vi "saveBuildHeader_III.vi"(6 "No. Averages":i32, 7 "Filtering":bool, 9 "wl 3":string="445", 10 "wl in":string="377", 11 "wl1":string="320") -> (2 "wavelengths":string[](array[string]), 3 "header":string[](array[string]))   [LabVIEW 2011]
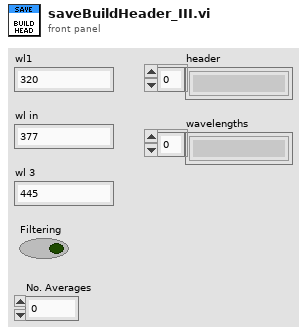
[diagram p1: front panel]
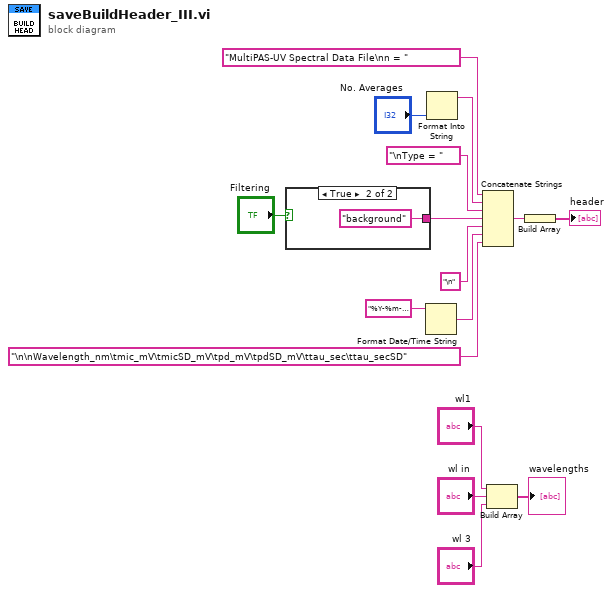
[diagram p0: block diagram]
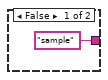
[diagram p2: hidden frame]
diagram:
  n1 = case shown="True" "Filtering" {
    tunnel: ["sample" "background"] -> w15
    frame False {
    }
    frame True {
    }
  }
  n2 = Format Date/Time String(time format string (%c)="%Y-%m-%d %H:%M:%S\t") -> (date/time string=w3:string)  [unwired: 2 in]
  n3 = Format Into String("No. Averages") -> (resulting string=w13:string)  [unwired: 3 in, 1 out]
  n4 = Concatenate Strings("MultiPAS-UV Spectral Data File\nn = ", w13, "\nType = " ("string"), w15, "\n" ("string"), w3, "\n\nWavelength_nm\tmic_mV\tmicSD_mV\tpd_mV\tpdSD_mV\ttau_sec\ttau_secSD" ("string")) -> (w5:string)
  n5 = Build Array("wl1", "wl in", "wl 3") -> (→"wavelengths":string[])
  n6 = Build Array(w5) -> (→"header":string[])
